vi "Initialize Daemon.vi"(8 "error in":errorcluster, 9 "Super Data Model":refnum<class "Super Data Model.lvclass">, 10 "transmission data unit":refnum<class "Transmission Data Unit.lvclass">, 11 "Serial Slave in":refnum<class "Serial Slave.lvclass">) -> (0 "error out":errorcluster, 3 "Serial Slave out":refnum<class "Serial Slave.lvclass">)   [LabVIEW 2013, in "Modbus Library - Advance.lvlib" / "Serial Slave.lvclass"]
doc: "This provides an interface for the slave to launch a protocol daemon."
uses:
  Serial Slave.lvclass
  Transmission Data Unit/Transmission Data Unit.lvclass
  Super Data Model/Super Data Model.lvclass
  Transmission Data Unit/Serial Interface/Serial Data Unit.lvclass
  Serial Slave.lvclass/Serial Slave.ctl
  Transmission Data Unit/Transmission Data Unit.lvclass/Transmission Data Unit.ctl
  Network Slave.lvclass
  Read VISA resource name.vi
  Read Baud Rate.vi
  Read Parity.vi
  Read Flow Control.vi
  Modbus Library - Advance.lvlib
  Serial Shared Components/Serial Shared Components.lvlib
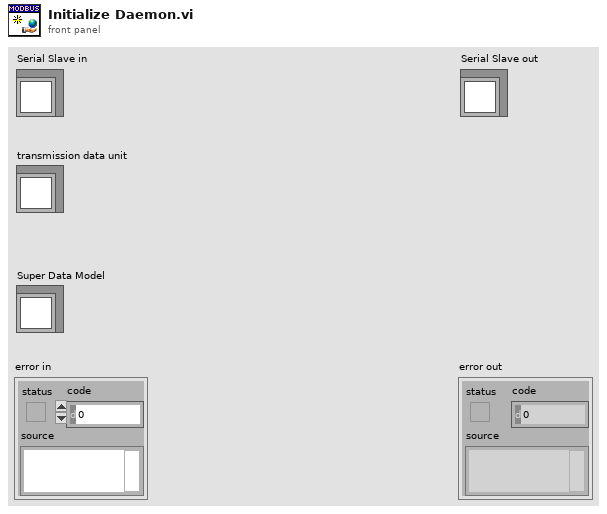
[diagram p1: front panel]
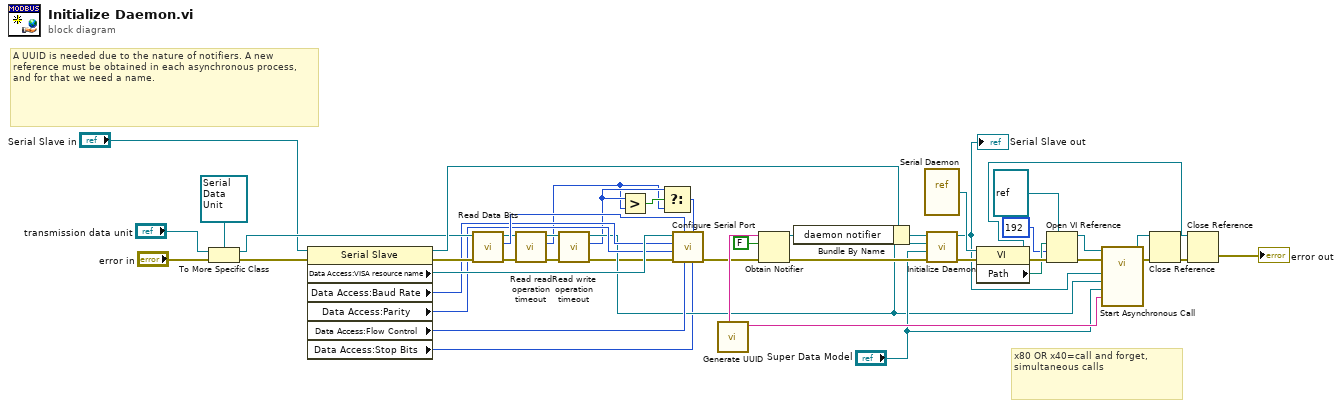
[diagram p0: block diagram]
diagram:
  # "x80 OR x40=call and forget, simultaneous calls"
  # "A UUID is needed due to the nature of notifiers. A new reference must be obtained in each asynchronous process, and for that we need a name."
  n1 = To More Specific Class(target class=refnum<class "Serial Data Unit.lvclass"> refnum ("Serial Data Unit in"), reference="transmission data unit", error in="error in") -> (specific class reference=w32:refnum<class "Serial Data Unit.lvclass">, error out=w34:errorcluster)
  n2 = property class="Serial Slave"(reference="Serial Slave in", error in=w34) -> (reference out=w36:refnum<class "Serial Slave.lvclass">, error out=w45:errorcluster, "Data Access:VISA resource name"=w30:refnum<visa-resource-name>, "Data Access:Baud Rate"=w28:u32, "Data Access:Parity"=w27:u16, "Data Access:Flow Control"=w26:u16, "Data Access:Stop Bits"=w1:u16)
  n3 = call-dynamic "Read Data Bits.vi"("error in (no error)"=w45, "Serial Data Unit in"=w32) -> ("error out"=w11:errorcluster, "data bits"=w29:u16, "Serial Data Unit out"=w14:refnum<class "Serial Data Unit.lvclass">)  [unwired: 7 in]
  n4 = call "Read read operation timeout.vi"("error in (no error)"=w11, "transmission data unit in"=w14) -> ("error out"=w12:errorcluster, "read operation timeout"=w8:i32, "transmission data unit out"=w15:refnum<class "Serial Data Unit.lvclass">)  [unwired: 7 in]
  n5 = call "Read write operation timeout.vi"("error in (no error)"=w12, "transmission data unit in"=w15) -> ("error out"=w6:errorcluster, "write operation timeout"=w9:i32, "transmission data unit out"=w13:refnum<class "Serial Data Unit.lvclass">)  [unwired: 7 in]
  n6 = Greater?(x=w9, y=w8) -> (0:w10:bool)
  n7 = Select(t=w9, s=w10, f=w8) -> (s? t:f=w7:i32)
  n8 = call "Configure Serial Port.vi"("Stop Bits"=w1, "Timeout"=w7, "Flow Control"=w26, "data bits"=w29, "error in (no error)"=w6, "Parity"=w27, "Baud Rate"=w28, "VISA Refnum in"=w30) -> ("error out"=w25:errorcluster)  [unwired: 3 in]
  n9 = call "Generate UUID.vi"() -> ("UUID"=w37:string)  [unwired: 11 in]
  n10 = Obtain Notifier(name (unnamed)=w37, notification data type=FALSE, error in (no error)=w25) -> (notifier out=w38:refnum<notifier>, error out=w22:errorcluster)  [unwired: 1 in, 1 out]
  n11 = Bundle By Name(cluster=w36, "daemon notifier"=w38) -> (w19:refnum<class "Serial Slave.lvclass">)
  n12 = vi-ref "Serial Daemon.vi"() -> (w44:refnum<vi>)
  n13 = call-parent "Initialize Daemon.vi"("error in"=w22, "Super Data Model"="Super Data Model", "transmission data unit"=w13, "network slave in"=w19) -> ("error out"=w21:errorcluster, "network slave out"=w20:refnum<class "Serial Slave.lvclass">)  [unwired: 6 in]
  "Serial Slave out" <- w20
  n14 = property class="VI"(reference=w44, error in=w21) -> (reference out=w2:refnum<vi>, error out=w43:errorcluster, "Path"=w42:path)
  n15 = Open VI Reference(type specifier VI Refnum (for type only)=refnum<vi> refnum, vi path=w42, options=192 ("x .or. y?"), error in (no error)=w43) -> (vi reference=w41:refnum<vi>, error out=w39:errorcluster)  [unwired: 2 in]
  n16 = call-by-ref "Start Asynchronous Call"(reference=w41, error in=w39, "UUID"=w37, "Super Data Model"="Super Data Model", "transmission data unit"=w13, "serial slave"=w20) -> (reference out=w3:refnum<vi>, error out=w31:errorcluster)  [unwired: 8 in]
  n17 = Close Reference(reference=w3, error in (no error)=w31) -> (error out=w4:errorcluster)
  n18 = Close Reference(reference=w2, error in (no error)=w4) -> (error out=→"error out":errorcluster)
